vi "Open FPGA Reference.vi"(0 "resource name":T1) -> (4 "FPGA VI Reference Out":refnum<k20>, 15 "error out":errorcluster)   [LabVIEW 2020, in "My Network Host v1.lvlib"]
uses:
  My Network Host v1.lvlib
  <vilib>/userDefined/Silver/nirio_resource_slv.ctl
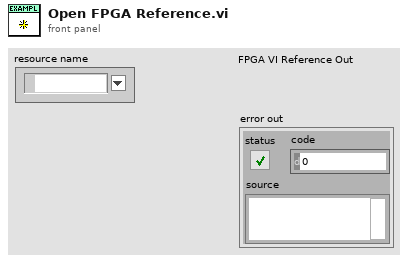
[diagram p1: front panel]
types:
  T1 = typedef "nirio_resource_slv.ctl" = tag
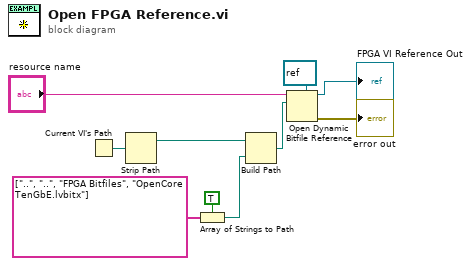
[diagram p0: block diagram]
diagram:
  n1 = Current VI's Path() -> (path=w6:path)
  n2 = Strip Path(path=w6) -> (stripped path=w5:path)  [unwired: 1 out]
  n3 = Array of Strings to Path(0:string[] ["..", "..", "FPGA Bitfiles", "OpenCore TenGbE.lvbitx"] ("array of strings"), 1:TRUE ("relative")) -> (2:w3:path)
  n4 = Build Path(base path=w5, name or relative path=w3) -> (appended path=w1:path)
  n5 = Open Dynamic Bitfile Reference(0:"resource name", 1:w1, 4:refnum<k20> refnum ("FPGA VI Reference Out")) -> (5:→"FPGA VI Reference Out":refnum<k20>, 8:→"error out":errorcluster)  [unwired: 2 in]
